vi "LabVIEW Object - Error Message Contains JSON Representation.vi"() -> ()   [LabVIEW 2017, in "Assertions.Tests.lvlib" / "Assert Equal.lvlib"]
uses:
  Assert Equal.lvlib
  src/Transparent Assertions/Constraints/IsEqual/Create.vi
  src/Transparent Assertions/Constraints/IsEqual/IsEqual.lvclass
  src/Transparent Assertions/Assertions/Assertions.lvlib
panel:
  out "error out":errorcluster
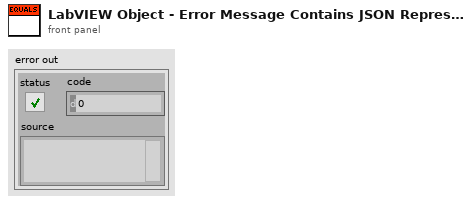
[diagram p1: front panel]
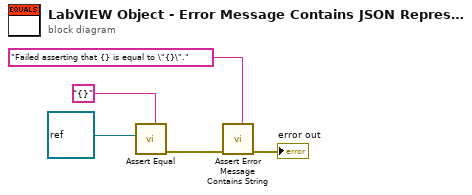
[diagram p0: block diagram]
diagram:
  n1 = call "Assert Equal.vi"("Expected"="{}", "Actual"=refnum<class> refnum ("LabVIEW Object")) -> ("error out"=w5:errorcluster)  [unwired: 9 in]
  n2 = call "Assert Error Message Contains String.vi"("Expected"="Failed asserting that {} is equal to \"{}\".", "error in (no error)"=w5) -> ("error out"=→"error out":errorcluster)  [unwired: 9 in]
